vi "Read_Sonar.vi"(0 "error in":errorcluster, 3 "node":string) -> (1 "error out":errorcluster, 4 "Point Cloud":T1)   [LabVIEW 2010]
doc: "This VI returns point cloud from the head sonar readings"
uses:
  ROS/Code/SubVIs/_ROSDirection.ctl
  ROS/Code/Console/Servers/ServerSubs/TopicDef.ctl
panel:
  out "Reply":string
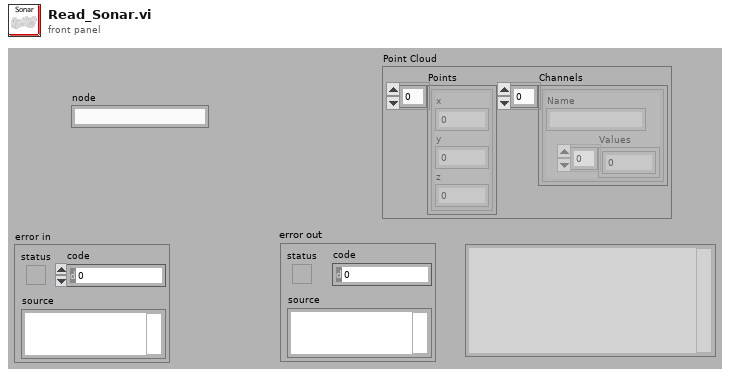
[diagram p1: front panel]
types:
  T1 = cluster{"Points":cluster{"x":sgl, "y":sgl, "z":sgl}[], "Channels":cluster{"Name":string, "Values":sgl[]}[]}
  T2 = typedef "TopicDef.ctl" = cluster{"Topic":string, "Type":string, "Action":T3, "Update (ms)":u16, "write queue":u16}
  T3 = typedef "_ROSDirection.ctl" = enum16{"Node", "Publisher", "Subscriber", "Service Client"}
  T4 = typedef "_ROSControl.ctl" = cluster{"topic port":u16, "Node":string, "topic":string, "type":string, "node port":u32, "error ":errorcluster, "Direction":T3, "APIs":string[], "Update (ms)":u16, "write queue":u16}
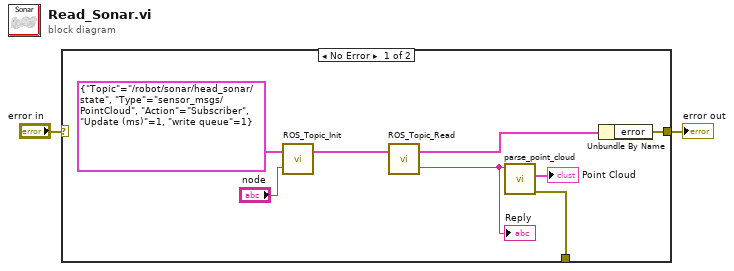
[diagram p0: block diagram]
diagram:
  n1 = case shown="No Error" "error in" {
    selector: "error in" -> [_ w11]
    tunnel: [w10 w11] -> w2
    tunnel: [w4 _] -> _
    frame No Error {
      n2 = call "ROS_Topic_Init.vi"("node"="node", "Definitions"=T2 {"Topic"="/robot/sonar/head_sonar/state", "Type"="sensor_msgs/PointCloud", "Action"=enum."Subscriber", "Update (ms)"=1, "write queue"=1}) -> ("ROS out"=w8:T4)  [unwired: 1 in]
      n3 = call "ROS_Topic_Read.vi"("ROS in"=w8) -> ("Reply"=w6:string, "ROS out"=w7:T4)  [unwired: 1 in]
      "Reply" <- w6
      n4 = call "parse_point_cloud.vi"("msg in"=w6) -> ("error out"=w4:errorcluster, "Point Cloud"=→"Point Cloud":T1)  [unwired: 3 in, 2 out]
      n5 = Unbundle By Name(w7) -> ("error"=w10:errorcluster)
    }
    frame Error {
    }
  }
  "error out" <- w2
